vi "1_2.vi"() -> ()   [LabVIEW 2023, in "2023.lvlib"]
uses:
  2023.lvlib
panel:
  out "Result":i32
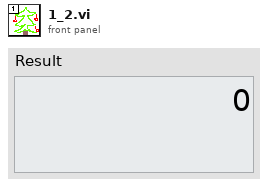
[diagram p1: front panel]
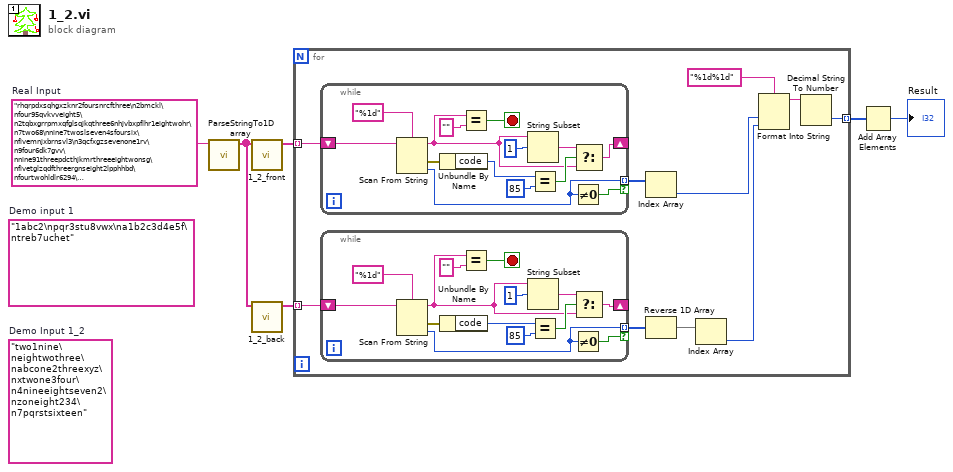
[diagram p0: block diagram]
diagram:
  (unwired) "1abc2\npqr3stu8vwx\na1b2c3d4e5f\ntreb7uchet"  # Demo input 1
  w3 = "rhqrpdxsqhgxzknr2foursnrcfthree\n2bmckl\nfour95qvkvveight5\n2tqbxgrrpmxqfglsqjkqthree6nhjvbxpflhr1eightwohr\n7two68\nnine7twoslseven4sfoursix\nfivemnjxbrnsvl3\n3qcfxgzsevenone1rv\n9four6dk7gvv\nnine91threepdcthjkmrthreeeightwonsg\nfivetglzqdfthreergnseight2lpphhbd\nfourtwohldlr6294\nqkvc7pvsv6rvsxlqzpjdjkd1eightthree\nonefourm5qpfvdnbs\nql8jbzzjpsdgmrjtngrkfdmcsix6eightsix\n8nl2\n5lfzqhgeightnine\nthree313eight2zcjnnmtnh\n4three77dgjzfj4five\nntr5sixfourznnljvqdr5one\nthreedlmnd98nineeighteight7\npzcnnbjjthreefmlf9znfnkdrjs\nflbdjkseven7338qxzbcsx6\nsix43fourthree2\none24hndgmz37mjqqm1\n4fiverlgtbr\n7hqtlxgngd15qkfl2th..."  # Real Input
  (unwired) "two1nine\neightwothree\nabcone2threexyz\nxtwone3four\n4nineeightseven2\nzoneight234\n7pqrstsixteen"  # Demo Input 1_2
  n1 = call "ParseStringTo1Darray.vi"("Copied Input From Advent Of Code Website"=w3) -> ("Formatted 1D String Array"=w2:string[])  [unwired: 10 in]
  n2 = call "1_2_front.vi"("Formatted 1D String Array"=w2) -> ("Array"=w5:string[])  [unwired: 10 in]
  n3 = call "1_2_back.vi"("Formatted 1D String Array"=w2) -> ("Array"=w4:string[])  [unwired: 10 in]
  n4 = for {
    tunnel: w5 -> [w16] mode=indexing
    tunnel: [w11] -> w6 mode=indexing
    tunnel: w4 -> [w8] mode=indexing
    n5 = while {
      shift-right: [w33] -> _
      shift-left: w16 -> [w44]
      tunnel: [w32] -> w15 mode=indexing if=w31
      stop <- w41 stop-if-true
      n6 = Scan From String(format string="%1d", input string=w44) -> (remaining string=w34:string, error out=w38:errorcluster, output 1=w32:i32)  [unwired: 3 in, 1 out]
      n7 = Unbundle By Name(w38) -> ("code"=w37:i32)
      n8 = Equal?(x=w34, y="") -> (x = y?=w41:bool)
      n9 = String Subset(string=w34, offset (0)=1) -> (substring=w35:string)  [unwired: 1 in]
      n10 = Equal?(x=w37, y=85 ("number 3")) -> (x = y?=w36:bool)
      n11 = Not Equal To 0?(x=w32) -> (x != 0?=w31:bool)
      n12 = Select(t=w35, s=w36, f=w34) -> (s? t:f=w33:string)
    }
    n13 = while {
      shift-right: [w19] -> _
      shift-left: w8 -> [w30]
      tunnel: [w18] -> w10 mode=indexing if=w17
      stop <- w27 stop-if-true
      n14 = Scan From String(format string="%1d", input string=w30) -> (remaining string=w20:string, error out=w24:errorcluster, output 1=w18:i32)  [unwired: 3 in, 1 out]
      n15 = Unbundle By Name(w24) -> ("code"=w23:i32)
      n16 = Equal?(x=w20, y="") -> (x = y?=w27:bool)
      n17 = String Subset(string=w20, offset (0)=1) -> (substring=w21:string)  [unwired: 1 in]
      n18 = Equal?(x=w23, y=85 ("number 3")) -> (x = y?=w22:bool)
      n19 = Not Equal To 0?(x=w18) -> (x != 0?=w17:bool)
      n20 = Select(t=w21, s=w22, f=w20) -> (s? t:f=w19:string)
    }
    n21 = Index Array(array=w15) -> (element=w13:i32)  [unwired: 1 in]
    n22 = Reverse 1D Array(array=w10) -> (reversed array=w9:i32[])
    n23 = Index Array(array=w9) -> (element=w7:i32)  [unwired: 1 in]
    n24 = Format Into String(format string="%1d%1d", w13, w7) -> (resulting string=w12:string)  [unwired: 2 in, 1 out]
    n25 = Decimal String To Number(string=w12) -> (number=w11:i32)  [unwired: 2 in, 1 out]
  }
  n26 = Add Array Elements(numeric array=w6) -> (sum=→"Result":i32)
